vi "XY Graph Get Selected Plots.vi"(8 "error in (no error)":errorcluster, 11 "XYGraph in":T1) -> (0 "error out":errorcluster, 1 "Selected Plots":i32[](array[numeric]), 2 "Selected Plot Names":string[](array[string]), 3 "XYGraph out":T1, 5 "Graph Name":string)   [LabVIEW 2019, in "XY Graph Add-Ons.lvlib"]
uses:
  XY Graph Add-Ons.lvlib
  XY Graph Refnum.ctl
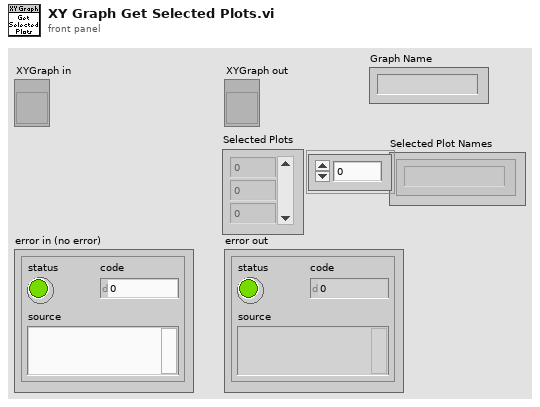
[diagram p1: front panel]
types:
  T1 = typedef "XY Graph Add-Ons.lvlib/XY Graph Refnum.ctl" = refnum<vi>
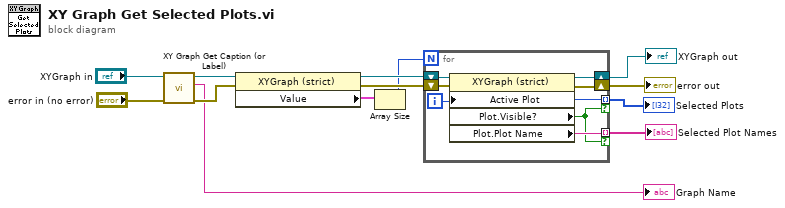
[diagram p0: block diagram]
diagram:
  n1 = call "XY Graph Get Caption (or Label).vi"("error in (no error)"="error in (no error)", "XYGraph in"="XYGraph in") -> ("error out"=w2:errorcluster, "Caption (or Label) Text"=→"Graph Name":string, "XYGraph out"=w4:T1)  [unwired: 7 in]
  n2 = property class="XYGraph (strict)"(reference=w4, error in=w2) -> (reference out=w12:T1, error out=w11:errorcluster, "Value"=w13:cluster{"X Array":dbl[], "Y Array":dbl[]}[])
  n3 = Array Size(array=w13) -> (size(s)=w7:i32)
  n4 = for {
    N: w7 -> [_]
    shift-right: [w19] -> w10
    shift-left: w12 -> [w20]
    tunnel: [w17] -> w8 mode=indexing if=w14
    shift-right: [w16] -> w9
    shift-left: w11 -> [w18]
    tunnel: [w15] -> w6 mode=indexing if=w14
    i -> [w17]
    n5 = property class="XYGraph (strict)"(reference=w20, error in=w18, "Active Plot"=w17) -> (reference out=w19:T1, error out=w16:errorcluster, "Plot.Visible?"=w14:bool, "Plot.Plot Name"=w15:string)
  }
  "XYGraph out" <- w10
  "error out" <- w9
  "Selected Plots" <- w8
  "Selected Plot Names" <- w6
